vi "Measurement Logic.vi"() -> ()   [LabVIEW 2021, in "Load Transient_Channel Ganging.lvlib"]
uses:
  Load Transient_Channel Ganging.lvlib
  <instrlib>/niDCPower/nidcpower.llb/niDCPower Source Mode.ctl
  <instrlib>/niDCPower/nidcpower.llb/niDCPower Output Function.ctl
  <instrlib>/niDCPower/nidcpower.llb/niDCPower Wait For Event - Event.ctl
  Users/upatel/OneDrive - Emerson/Desktop/S!/source/channel ganging/shared subVIs/ctl/NIDCPower_channel_ganging - ctl - channel mode.ctl
  Measurement Results.ctl
  <vilib>/Plug-In SDKs/Measurements/Measure Call Context/Measure Call Context.lvclass
  Measurement Configuration.ctl
panel:
  out "measurement results":T1
  in  "measurement configuration":T2={"Source system configuration"=enum."Parallel", "Source voltage level range"=1.2, "Source limit symmetry"=enum."Asymmetric", "Source current limit range"=32.0, "Source current limit low"=64.0, "Source current limit high"=64.0, "Load system configuration"=enum."Series", "Source transient response"=-32, "Source sense"=-64, "Source voltage level"=-64.0, "Source master resource name"="Lorem ipsum dolor sit", "Load master resource name"="Lorem ipsum dolor sit", "Source slave resource names"=["", ""], "Load slave resource names"=["", ""], "Source voltage gain bandwidth"=1.0, "Source voltage compensation frequency"=1.0, "Source voltage pole-zero ratio"=2.0, "Load sample rate"=1800000.0, "Load current level range"=80.0, "Load limit symmetry"=enum."Symmetric", "Load voltage limit range"=6.0, "Load voltage limit low"=0.0, "Load voltage limit high"=inf, "Load transient response"=1038, "Load sense"=1009, "Load current set point 1"=4.0, "Load current set point 2"=14.0, "Load current gain bandwidth"=14000.0, "Load current compensation frequency"=180000.0, "Load current pole-zero ratio"=0.3, "DUT setup time"=1.0, "Nominal output voltage"=1.0, "Dwell time"=0.005} {"Load sense" items=["Local"=1008, "Remote"=1009]; "Load transient response" items=["Slow"=1041, "Normal"=1038, "Fast"=1039, "Custom"=1042]; "Load voltage limit high" format="%#_6p"; "Load voltage limit low" format="%#_6p"; "Load voltage limit range" format="%#_6p"; "Load current level range" format="%#_6p"; "Source sense" items=["Local"=1008, "Remote"=1009]; "Source transient response" items=["Slow"=1041, "Normal"=1038, "Fast"=1039, "Custom"=1042]; "Source current limit low" format="%#_6p"}
  out "measure call context out":refnum<class "Measure Call Context.lvclass">
  in  "measure call context in":refnum<class "Measure Call Context.lvclass">
  out "error out":errorcluster
  in  "error in":errorcluster
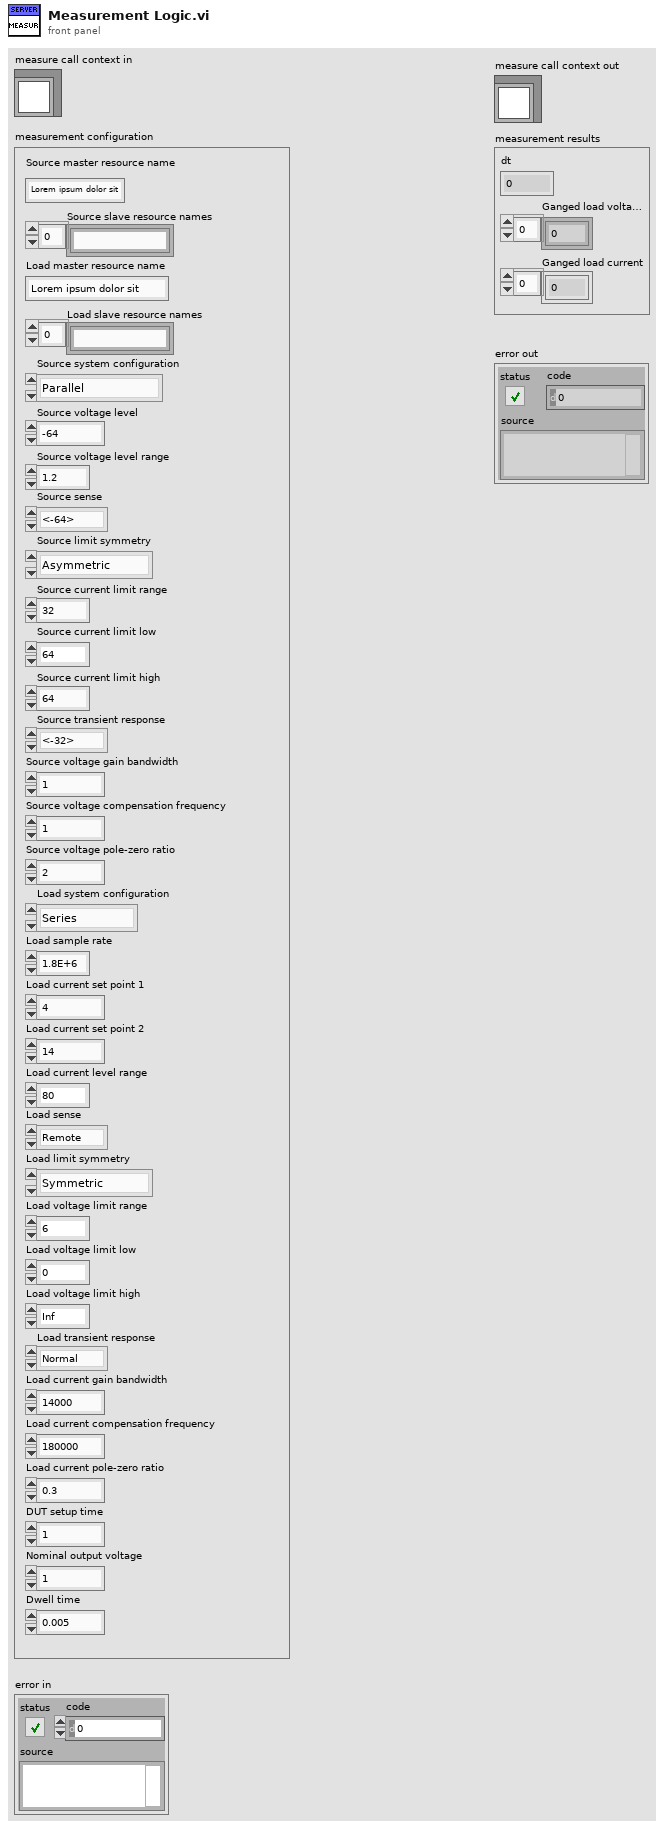
[diagram p1: front panel]
types:
  T1 = typedef "Load Transient_Channel Ganging.lvlib/Measurement Results.ctl" = cluster{"dt":dbl, "Ganged load voltages":dbl[], "Ganged load current":dbl[]}
  T2 = typedef "Load Transient_Channel Ganging.lvlib/Measurement Configuration.ctl" = cluster{"Source system configuration":enum32{"Series", "Parallel", "Manual"}, "Source voltage level range":dbl, "Source limit symmetry":enum32{"Symmetric", "Asymmetric"}, "Source current limit range":dbl, "Source current limit low":dbl, "Source current limit high":dbl, "Load system configuration":enum32{"Series", "Parallel", "Manual"}, "Source transient response":i32, "Source sense":i32, "Source voltage level":dbl, "Source master resource name":string, "Load master resource name":string, "Source slave resource names":string[], "Load slave resource names":string[], "Source voltage gain bandwidth":dbl, "Source voltage compensation frequency":dbl, "Source voltage pole-zero ratio":dbl, "Load sample rate":dbl, "Load current level range":dbl, "Load limit symmetry":enum32{"Symmetric", "Asymmetric"}, "Load voltage limit range":dbl, "Load voltage limit low":dbl, "Load voltage limit high":dbl, "Load transient response":i32, "Load sense":i32, "Load current set point 1":dbl, "Load current set point 2":dbl, "Load current gain bandwidth":dbl, "Load current compensation frequency":dbl, "Load current pole-zero ratio":dbl, "DUT setup time":dbl, "Nominal output voltage":dbl, "Dwell time":dbl}
  T3 = typedef "NIDCPower_channel_ganging - ctl - channel mode.ctl" = enum32{"Master", "Slave", "Slave - Inverted"}
  T4 = typedef "niDCPower Wait For Event - Event.ctl" = i32
  T5 = typedef "niDCPower Output Function.ctl" = i32
  T6 = typedef "niDCPower Source Mode.ctl" = i32
  T7 = typedef "NIDCPower_channel_ganging - ctl - channel def.ctl" = cluster{"resource name":refnum<k15>, "channels":string, "Channel Mode":T3}
  T8 = typedef "NIDCPower_channel_ganging - ctl - ganged session.ctl" = cluster{"Ganged Config":T9, "Session List":refnum<k15>[], "Session Mode":T3[], "Channel":string[]}
  T9 = typedef "NIDCPower_channel_ganging - ctl - ganged config.ctl" = enum32{"Series", "Parallel", "Manual"}
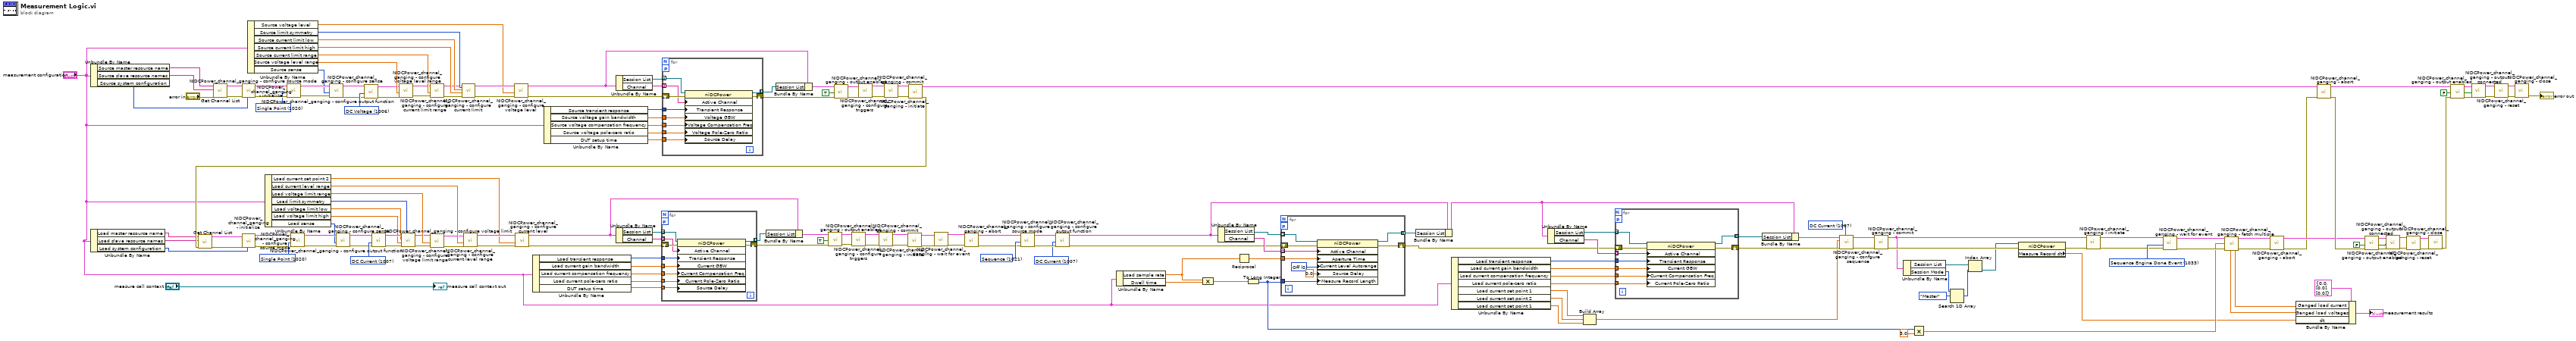
[diagram p0: block diagram]
diagram:
  w30 = FALSE ("output enabled")
  w29 = FALSE ("output enabled")
  w44 = T4 1033 items=["Source Complete Event"=1030, "Measure Complete Event"=1031, "Sequence Iteration Complete Event"=1032, "Sequence Engine Done Event"=1033, "Pulse Complete Event"=1051, "Ready For Pulse Trigger Event"=1052] ("event")
  w60 = T5 1007 items=["DC Voltage"=1006, "DC Current"=1007, "Pulse Voltage"=1049, "Pulse Current"=1050] ("output function")
  w83 = T6 1021 items=["Single Point"=1020, "Sequence"=1021] ("source mode")
  w82 = T5 1007 items=["DC Voltage"=1006, "DC Current"=1007, "Pulse Voltage"=1049, "Pulse Current"=1050] ("output function")
  w143 = T5 1007 items=["DC Voltage"=1006, "DC Current"=1007, "Pulse Voltage"=1049, "Pulse Current"=1050] ("output function")
  w156 = T5 1006 items=["DC Voltage"=1006, "DC Current"=1007, "Pulse Voltage"=1049, "Pulse Current"=1050] ("output function")
  w175 = T6 1020 items=["Single Point"=1020, "Sequence"=1021] ("source mode")
  w176 = T6 1020 items=["Single Point"=1020, "Sequence"=1021] ("source mode")
  n1 = Unbundle By Name("measurement configuration") -> ("Source master resource name"=w102:string, "Source slave resource names"=w101:string[], "Source system configuration"=w158:enum32{"Series", "Parallel", "Manual"})
  n2 = Unbundle By Name("measurement configuration") -> ("Load master resource name"=w98:string, "Load slave resource names"=w97:string[], "Load system configuration"=w157:enum32{"Series", "Parallel", "Manual"})
  n3 = call "Get Channel List.vi"("error in (no error)"="error in", "Slave resource names"=w101, "Master resouce name"=w102) -> ("error out"=w103:errorcluster, "Channel List"=w104:T7[])  [unwired: 7 in]
  n4 = call "NIDCPower_channel_ganging - initialize.vi"("Ganged Config"=w158, "error in (no error)"=w103, "Channel List"=w104) -> ("error out"=w177:errorcluster, "Ganged Session Out"=w178:T8)  [unwired: 7 in]
  n5 = Unbundle By Name("measurement configuration") -> ("Source voltage level"=w86:dbl, "Source limit symmetry"=w164:enum32{"Symmetric", "Asymmetric"}, "Source current limit low"=w165:dbl, "Source current limit high"=w166:dbl, "Source current limit range"=w167:dbl, "Source voltage level range"=w168:dbl, "Source sense"=w105:i32)
  n6 = Unbundle By Name("measurement configuration") -> ("Load current set point 2"=w107:dbl, "Load current level range"=w159:dbl, "Load voltage limit range"=w160:dbl, "Load limit symmetry"=w163:enum32{"Symmetric", "Asymmetric"}, "Load voltage limit low"=w162:dbl, "Load voltage limit high"=w161:dbl, "Load sense"=w106:i32)
  n7 = call "NIDCPower_channel_ganging - configure source mode.vi"("error in (no error)"=w177, "source mode"=w176, "Ganged Session In"=w178) -> ("error out"=w141:errorcluster, "Ganged Session Out"=w142:T8)  [unwired: 7 in]
  n8 = call "NIDCPower_channel_ganging - configure sense.vi"("error in (no error)"=w141, "sense"=w105, "Ganged Session In"=w142) -> ("error out"=w139:errorcluster, "Ganged Session Out"=w140:T8)  [unwired: 7 in]
  n9 = call "NIDCPower_channel_ganging - configure output function.vi"("error in (no error)"=w139, "output function"=w156, "Ganged Session In"=w140) -> ("error out"=w137:errorcluster, "Ganged Session Out"=w138:T8)  [unwired: 7 in]
  n10 = call "NIDCPower_channel_ganging - configure voltage level range.vi"("error in (no error)"=w137, "voltage level range"=w168, "Ganged Session In"=w138) -> ("error out"=w152:errorcluster, "Ganged Session Out"=w155:T8)  [unwired: 7 in]
  n11 = call "NIDCPower_channel_ganging - configure current limit range.vi"("error in (no error)"=w152, "current limit range"=w167, "Ganged Session In"=w155) -> ("error out"=w151:errorcluster, "Ganged Session Out"=w154:T8)  [unwired: 7 in]
  n12 = call "NIDCPower_channel_ganging - configure current limit.vi"("Limit Symmetry"=w164, "error in (no error)"=w151, "Current limit/hi"=w166, "Current limit lo"=w165, "Ganged Session In"=w154) -> ("error out"=w150:errorcluster, "Ganged Session Out"=w153:T8)  [unwired: 5 in]
  n13 = call "NIDCPower_channel_ganging - configure voltage level.vi"("error in (no error)"=w150, "voltage level"=w86, "Ganged Session In"=w153) -> ("error out"=w115:errorcluster, "Ganged Session Out"=w49:T8)  [unwired: 7 in]
  n14 = Unbundle By Name("measurement configuration") -> ("Load transient response"=w95:i32, "Load current gain bandwidth"=w89:dbl, "Load current compensation frequency"=w88:dbl, "Load current pole-zero ratio"=w87:dbl, "DUT setup time"=w94:dbl)
  n15 = Unbundle By Name("measurement configuration") -> ("Source transient response"=w96:i32, "Source voltage gain bandwidth"=w92:dbl, "Source voltage compensation frequency"=w91:dbl, "Source voltage pole-zero ratio"=w90:dbl, "DUT setup time"=w93:dbl)
  n16 = Unbundle By Name(w49) -> ("Session List"=w113:refnum<k15>[], "Channel"=w112:string[])
  n17 = for {
    tunnel: [w189] -> w48 mode=indexing
    shift-right: [w187] -> w114
    shift-left: w115 -> [w188]
    workers-P: _ -> [_]
    tunnel: w113 -> [w186] mode=indexing
    tunnel: w112 -> [w185] mode=indexing
    tunnel: w96 -> [w184]
    tunnel: w93 -> [w183]
    tunnel: w92 -> [w182]
    tunnel: w91 -> [w181]
    tunnel: w90 -> [w180]
    n18 = property class="niDCPower"(reference=w186, error in=w188, "Active Channel"=w185, "Transient Response"=w184, "Voltage GBW"=w182, "Voltage Compensation Freq"=w181, "Voltage Pole-Zero Ratio"=w180, "Source Delay"=w183) -> (reference out=w189:refnum<k15>, error out=w187:errorcluster)
  }
  n19 = Bundle By Name(cluster=w49, "Session List"=w48) -> (w47:T8)
  n20 = call "NIDCPower_channel_ganging - output enabled.vi"("error in (no error)"=w114, "output enabled"=TRUE, "Ganged Session In"=w47) -> ("error out"=w118:errorcluster, "Ganged Session Out"=w119:T8)  [unwired: 7 in]
  n21 = call "NIDCPower_channel_ganging - configure triggers.vi"("error in (no error)"=w118, "Ganged Session In"=w119) -> ("error out"=w116:errorcluster, "Ganged Session Out"=w117:T8)  [unwired: 8 in]
  n22 = call "NIDCPower_channel_ganging - commit.vi"("error in (no error)"=w116, "Ganged Session In"=w117) -> ("error out"=w125:errorcluster, "Ganged Session Out"=w124:T8)  [unwired: 8 in]
  n23 = call "NIDCPower_channel_ganging - initiate.vi"("error in (no error)"=w125, "Ganged Session In"=w124) -> ("error out"=w126:errorcluster, "Ganged Session Out"=w18:T8)  [unwired: 8 in]
  n24 = call "Get Channel List.vi"("error in (no error)"=w126, "Slave resource names"=w97, "Master resouce name"=w98) -> ("error out"=w100:errorcluster, "Channel List"=w99:T7[])  [unwired: 7 in]
  n25 = call "NIDCPower_channel_ganging - initialize.vi"("Ganged Config"=w157, "error in (no error)"=w100, "Channel List"=w99) -> ("error out"=w174:errorcluster, "Ganged Session Out"=w173:T8)  [unwired: 7 in]
  n26 = call "NIDCPower_channel_ganging - configure source mode.vi"("error in (no error)"=w174, "source mode"=w175, "Ganged Session In"=w173) -> ("error out"=w135:errorcluster, "Ganged Session Out"=w136:T8)  [unwired: 7 in]
  n27 = call "NIDCPower_channel_ganging - configure sense.vi"("error in (no error)"=w135, "sense"=w106, "Ganged Session In"=w136) -> ("error out"=w133:errorcluster, "Ganged Session Out"=w134:T8)  [unwired: 7 in]
  n28 = call "NIDCPower_channel_ganging - configure output function.vi"("error in (no error)"=w133, "output function"=w143, "Ganged Session In"=w134) -> ("error out"=w171:errorcluster, "Ganged Session Out"=w172:T8)  [unwired: 7 in]
  n29 = call "NIDCPower_channel_ganging - configure voltage limit.vi"("Limit Symmetry"=w163, "error in (no error)"=w171, "voltage limit/hi"=w161, "voltage limit lo"=w162, "Ganged Session In"=w172) -> ("error out"=w148:errorcluster, "Ganged Session Out"=w149:T8)  [unwired: 5 in]
  n30 = call "NIDCPower_channel_ganging - configure voltage limit range.vi"("error in (no error)"=w148, "voltage level range"=w160, "Ganged Session In"=w149) -> ("error out"=w146:errorcluster, "Ganged Session Out"=w147:T8)  [unwired: 7 in]
  n31 = call "NIDCPower_channel_ganging - configure current level range.vi"("error in (no error)"=w146, "current level range"=w159, "Ganged Session In"=w147) -> ("error out"=w144:errorcluster, "Ganged Session Out"=w145:T8)  [unwired: 7 in]
  n32 = call "NIDCPower_channel_ganging - configure current level.vi"("error in (no error)"=w144, "current level"=w107, "Ganged Session In"=w145) -> ("error out"=w111:errorcluster, "Ganged Session Out"=w52:T8)  [unwired: 7 in]
  n33 = Unbundle By Name(w52) -> ("Session List"=w109:refnum<k15>[], "Channel"=w108:string[])
  n34 = for {
    tunnel: [w199] -> w50 mode=indexing
    shift-right: [w197] -> w110
    shift-left: w111 -> [w198]
    workers-P: _ -> [_]
    tunnel: w109 -> [w196] mode=indexing
    tunnel: w108 -> [w195] mode=indexing
    tunnel: w95 -> [w194]
    tunnel: w94 -> [w193]
    tunnel: w89 -> [w192]
    tunnel: w88 -> [w191]
    tunnel: w87 -> [w190]
    n35 = property class="niDCPower"(reference=w196, error in=w198, "Active Channel"=w195, "Transient Response"=w194, "Current GBW"=w192, "Current Compensation Freq"=w191, "Current Pole-Zero Ratio"=w190, "Source Delay"=w193) -> (reference out=w199:refnum<k15>, error out=w197:errorcluster)
  }
  n36 = Bundle By Name(cluster=w52, "Session List"=w50) -> (w51:T8)
  n37 = call "NIDCPower_channel_ganging - output enabled.vi"("error in (no error)"=w110, "output enabled"=TRUE, "Ganged Session In"=w51) -> ("error out"=w122:errorcluster, "Ganged Session Out"=w123:T8)  [unwired: 7 in]
  n38 = call "NIDCPower_channel_ganging - configure triggers.vi"("error in (no error)"=w122, "Ganged Session In"=w123) -> ("error out"=w120:errorcluster, "Ganged Session Out"=w121:T8)  [unwired: 8 in]
  n39 = call "NIDCPower_channel_ganging - commit.vi"("error in (no error)"=w120, "Ganged Session In"=w121) -> ("error out"=w131:errorcluster, "Ganged Session Out"=w132:T8)  [unwired: 8 in]
  n40 = call "NIDCPower_channel_ganging - initiate.vi"("error in (no error)"=w131, "Ganged Session In"=w132) -> ("error out"=w129:errorcluster, "Ganged Session Out"=w130:T8)  [unwired: 8 in]
  n41 = call "NIDCPower_channel_ganging - wait for event.vi"("error in (no error)"=w129, "Ganged Session in"=w130) -> ("error out"=w127:errorcluster, "Ganged Session Out"=w128:T8)  [unwired: 8 in]
  n42 = call "NIDCPower_channel_ganging - abort.vi"("error in (no error)"=w127, "Ganged Session In"=w128) -> ("error out"=w81:errorcluster, "Ganged Session Out"=w80:T8)  [unwired: 8 in]
  n43 = call "NIDCPower_channel_ganging - configure source mode.vi"("error in (no error)"=w81, "source mode"=w83, "Ganged Session In"=w80) -> ("error out"=w85:errorcluster, "Ganged Session Out"=w84:T8)  [unwired: 7 in]
  n44 = call "NIDCPower_channel_ganging - configure output function.vi"("error in (no error)"=w85, "output function"=w82, "Ganged Session In"=w84) -> ("error out"=w77:errorcluster, "Ganged Session Out"=w54:T8)  [unwired: 7 in]
  n45 = Unbundle By Name("measurement configuration") -> ("Load sample rate"=w74:dbl, "Dwell time"=w73:dbl)
  n46 = Compound Arithmetic op=MULTIPLY(w74, w73) -> (w75:dbl)
  n47 = Unbundle By Name(w54) -> ("Session List"=w79:refnum<k15>[], "Channel"=w78:string[])
  n48 = Reciprocal(x=w74) -> (1/x=w76:dbl)
  n49 = To Long Integer(number=w75) -> (32bit integer=w15:i32)
  n50 = for {
    tunnel: [w208] -> w55 mode=indexing
    shift-right: [w206] -> w66
    shift-left: w77 -> [w207]
    workers-P: _ -> [_]
    tunnel: w79 -> [w205] mode=indexing
    tunnel: w78 -> [w204] mode=indexing
    tunnel: w76 -> [w203]
    tunnel: w15 -> [w201]
    w200 = 0 items=["Off", "On"] ("Source:DC Current:Current Level Autorange")
    n51 = property class="niDCPower"(reference=w205, error in=w207, "Active Channel"=w204, "Aperture Time"=w203, "Current Level Autorange"=w200, "Source Delay"=0.0 ("Source:Advanced:Source Delay"), "Measure Record Length"=w201) -> (reference out=w208:refnum<k15>, error out=w206:errorcluster)
  }
  n52 = Bundle By Name(cluster=w54, "Session List"=w55) -> (w53:T8)
  n53 = Unbundle By Name("measurement configuration") -> ("Load transient response"=w70:i32, "Load current gain bandwidth"=w69:dbl, "Load current compensation frequency"=w68:dbl, "Load current pole-zero ratio"=w67:dbl, "Load current set point 1"=w64:dbl, "Load current set point 2"=w63:dbl, "Load current set point 1"=w62:dbl)
  n54 = Unbundle By Name(w53) -> ("Session List"=w72:refnum<k15>[], "Channel"=w71:string[])
  n55 = Build Array(w64, w63, w62) -> (w61:dbl[])
  n56 = for {
    tunnel: [w217] -> w57 mode=indexing
    shift-right: [w215] -> w65
    shift-left: w66 -> [w216]
    workers-P: _ -> [_]
    tunnel: w72 -> [w214] mode=indexing
    tunnel: w71 -> [w213] mode=indexing
    tunnel: w70 -> [w212]
    tunnel: w69 -> [w211]
    tunnel: w68 -> [w210]
    tunnel: w67 -> [w209]
    n57 = property class="niDCPower"(reference=w214, error in=w216, "Active Channel"=w213, "Transient Response"=w212, "Current GBW"=w211, "Current Compensation Freq"=w210, "Current Pole-Zero Ratio"=w209) -> (reference out=w217:refnum<k15>, error out=w215:errorcluster)
  }
  n58 = Bundle By Name(cluster=w53, "Session List"=w57) -> (w56:T8)
  n59 = call "NIDCPower_channel_ganging - confgure sequence.vi"("output function"=w60, "error in (no error)"=w65, "Values"=w61, "Ganged Session In"=w56) -> ("error out"=w59:errorcluster, "Ganged Session Out"=w58:T8)  [unwired: 6 in]
  n60 = call "NIDCPower_channel_ganging - commit.vi"("error in (no error)"=w59, "Ganged Session In"=w58) -> ("error out"=w46:errorcluster, "Ganged Session Out"=w45:T8)  [unwired: 8 in]
  n61 = Unbundle By Name(w45) -> ("Session List"=w13:refnum<k15>[], "Session Mode"=w12:T3[])
  n62 = Multiply(x=w15, y=3.0) -> (x*y=w17:dbl)
  n63 = Search 1D Array(1D array=w12, element=NIDCPower_channel_ganging_-_ctl_-_channel_mode."Master") -> (index of element=w10:i32)  [unwired: 1 in]
  n64 = Index Array(array=w13, index=w10) -> (element=w14:refnum<k15>)
  n65 = property class="niDCPower"(reference=w14, error in=w46) -> (error out=w42:errorcluster, "Measure Record dt"=w1:dbl)  [unwired: 1 out]
  n66 = call "NIDCPower_channel_ganging - initiate.vi"("error in (no error)"=w42, "Ganged Session In"=w45) -> ("error out"=w41:errorcluster, "Ganged Session Out"=w43:T8)  [unwired: 8 in]
  n67 = call "NIDCPower_channel_ganging - wait for event.vi"("error in (no error)"=w41, "event"=w44, "Ganged Session in"=w43) -> ("error out"=w39:errorcluster, "Ganged Session Out"=w40:T8)  [unwired: 7 in]
  n68 = call "NIDCPower_channel_ganging - fetch multiple.vi"("Ganged Session In"=w40, "Count"=w17, "error in (no error)"=w39) -> ("Ganged Voltage Measurement"=w3:dbl[], "Ganged Current Measurement"=w2:dbl[], "Ganged Session Out"=w20:T8, "error out"=w19:errorcluster)  [unwired: 5 in, 4 out]
  n69 = call "NIDCPower_channel_ganging - abort.vi"("error in (no error)"=w19, "Ganged Session In"=w20) -> ("error out"=w4:errorcluster, "Ganged Session Out"=w35:T8)  [unwired: 8 in]
  n70 = Bundle By Name(cluster=T1 {"dt"=0.0, "Ganged load voltages"=[0.0], "Ganged load current"=[0.0]} ("measurement results"), "Ganged load current"=w2, "Ganged load voltages"=w3, "dt"=w1) -> (→"measurement results":T1)
  n71 = call "NIDCPower_channel_ganging - abort.vi"("error in (no error)"=w4, "Ganged Session In"=w18) -> ("error out"=w38:errorcluster, "Ganged Session Out"=w31:T8)  [unwired: 8 in]
  n72 = call "NIDCPower_channel_ganging - output enabled.vi"("error in (no error)"=w38, "output enabled"=w30, "Ganged Session In"=w35) -> ("error out"=w36:errorcluster, "Ganged Session Out"=w37:T8)  [unwired: 7 in]
  n73 = call "NIDCPower_channel_ganging - output connected.vi"("error in (no error)"=w36, "output enabled"=w30, "Ganged Session In"=w37) -> ("error out"=w28:errorcluster, "Ganged Session Out"=w27:T8)  [unwired: 7 in]
  n74 = call "NIDCPower_channel_ganging - reset.vi"("error in (no error)"=w28, "Ganged Session In"=w27) -> ("error out"=w25:errorcluster, "Ganged Session Out"=w26:T8)  [unwired: 8 in]
  n75 = call "NIDCPower_channel_ganging - close.vi"("error in (no error)"=w25, "Ganged Session In"=w26) -> ("error out"=w32:errorcluster)  [unwired: 9 in]
  n76 = call "NIDCPower_channel_ganging - output enabled.vi"("error in (no error)"=w32, "output enabled"=w29, "Ganged Session In"=w31) -> ("error out"=w34:errorcluster, "Ganged Session Out"=w33:T8)  [unwired: 7 in]
  n77 = call "NIDCPower_channel_ganging - output connected.vi"("error in (no error)"=w34, "output enabled"=w29, "Ganged Session In"=w33) -> ("error out"=w23:errorcluster, "Ganged Session Out"=w24:T8)  [unwired: 7 in]
  n78 = call "NIDCPower_channel_ganging - reset.vi"("error in (no error)"=w23, "Ganged Session In"=w24) -> ("error out"=w21:errorcluster, "Ganged Session Out"=w22:T8)  [unwired: 8 in]
  n79 = call "NIDCPower_channel_ganging - close.vi"("error in (no error)"=w21, "Ganged Session In"=w22) -> ("error out"=→"error out":errorcluster)  [unwired: 9 in]
  "measure call context out" <- "measure call context in"
